vi "ClearInterlock.vi"(11 "Station":string) -> ()   [LabVIEW 2020]
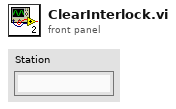
[diagram p1: front panel]
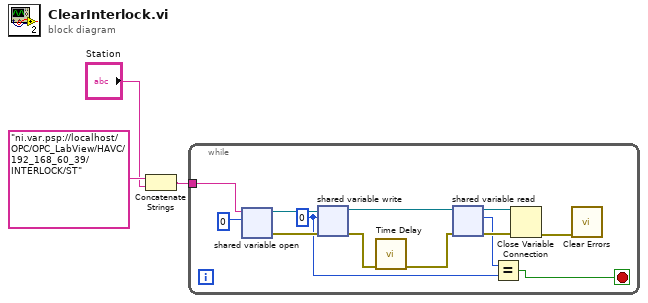
[diagram p0: block diagram]
diagram:
  n1 = Concatenate Strings("ni.var.psp://localhost/OPC/OPC_LabView/HAVC/192_168_60_39/INTERLOCK/ST" ("string"), "Station") -> (w3:string)
  n2 = while {
    tunnel: w3 -> [w4]
    stop <- w5 stop-if-true
    w6 = 0 ("data in")
    n3 = shared-variable-open(w4, 0) -> (w15:refnum<k21>, w14:errorcluster)  [unwired: 2 in]
    n4 = shared-variable-write(w15, w14, w6) -> (w9:refnum<k21>, w12:errorcluster)
    n5 = call "Time Delay"("error in (no error)"=w12) -> ("error out"=w10:errorcluster)  [unwired: 10 in]
    n6 = shared-variable-read(w9, w10) -> (w8:refnum<k21>, w11:errorcluster, w7:i32)  [unwired: 1 out]
    n7 = Equal?(x=w7, y=w6) -> (x = y?=w5:bool)
    n8 = Close Variable Connection(8:w11, 11:w8) -> (0:w13:errorcluster)
    n9 = call <vilib>:"Clear Errors.vi"("error in (no error)"=w13) -> ()  [unwired: 5 in, 2 out]
  }
